vi "一维积分.vi"() -> ()   [LabVIEW 2018]
uses:
  <vilib>/Analysis/8numeric.llb/1D Quadrature (Formula).vi
  <vilib>/Analysis/NI_AALPro.lvlib
panel:
  in  "停止":bool
  out "积分结果":dbl
  in  "函数":string
  in  "积分下限":dbl
  in  "积分上限":dbl
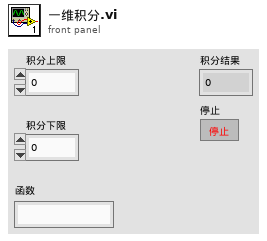
[diagram p1: front panel]
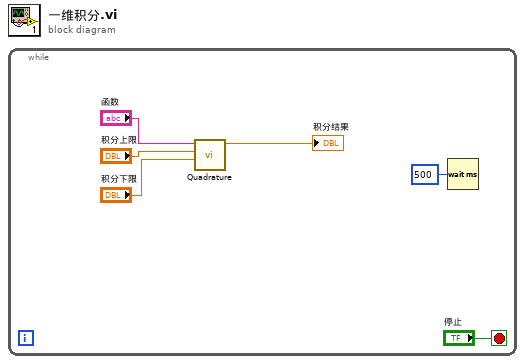
[diagram p0: block diagram]
diagram:
  n1 = while {
    stop <- "停止" stop-if-true
    n2 = call-poly <vilib>:"Quadrature.vi"("lower limit"="积分下限", "upper limit"="积分上限", "integrand"="函数") -> ("result"=→"积分结果":dbl)  [unwired: 7 in, 1 out]
    n3 = Wait (ms)(milliseconds to wait=u32 500 ("等待时间（毫秒）")) -> ()  [unwired: 1 out]
  }
